vi "Manipulate frame size.vi"(8 "error in (no error)":errorcluster, 10 "Value":u16, 11 "Frame Size":refnum<vi>) -> (0 "error out":errorcluster, 3 "Updated frame size":T1=200 items=["100X100"=100, "128X128"=128, "200X200"=200, "256X256"=256, "512X512"=512, "1024x1024"=1024, "2048x2048"=2048])   [LabVIEW 2020]
uses:
  Typedefs/Frame Size.ctl
  3abac306-aade-448e-83a5-8b61187ab33a.vi
  <vilib>/Comparison/Equal/Equal Functor/Equal Functor.lvclass
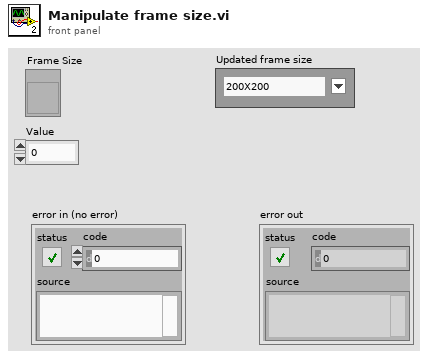
[diagram p1: front panel]
types:
  T1 = typedef "Frame Size.ctl" = u16
  T2 = typedef "LVStringsAndValuesArrayTypeDef_U16.ctl" = cluster{"String":string, "Value":u16}[]
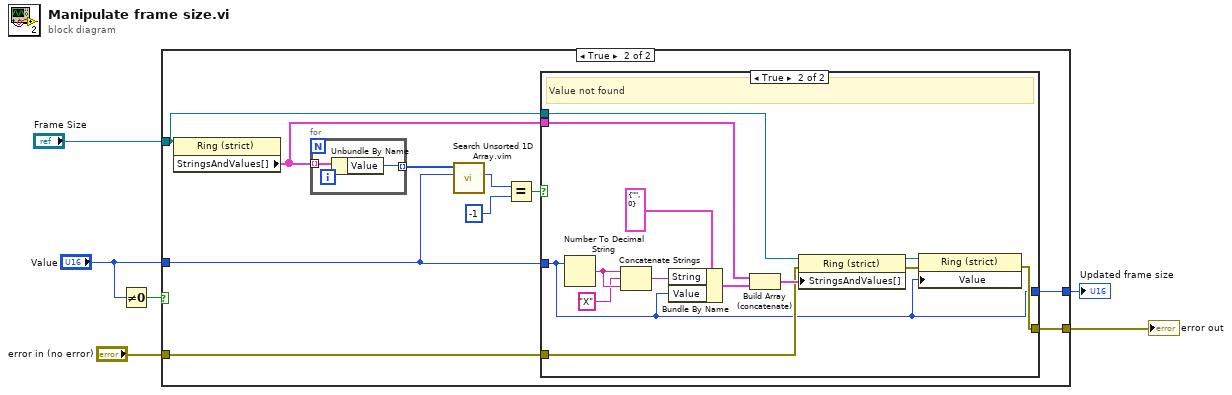
[diagram p0: block diagram]
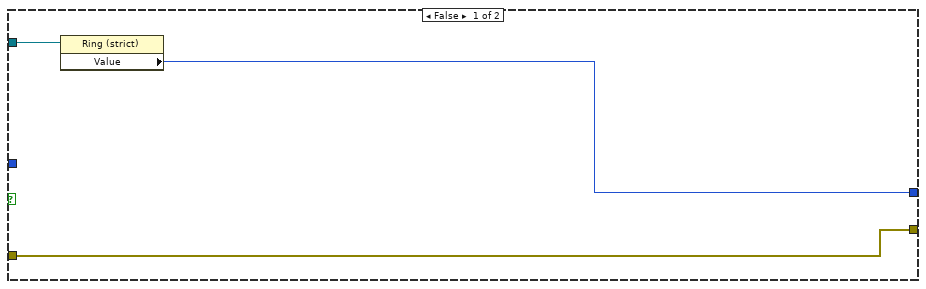
[diagram p2: hidden frame]
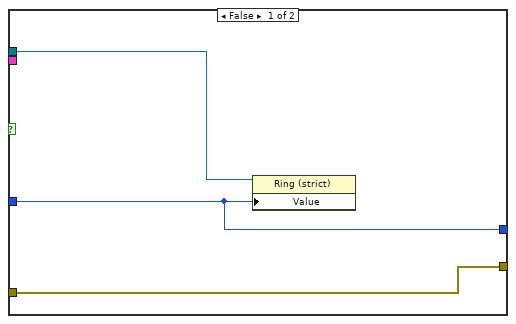
[diagram p3: hidden frame]
diagram:
  n1 = Not Equal To 0?(x="Value") -> (x != 0?=w4:bool)
  n2 = case shown="True" w4 {
    tunnel: "Frame Size" -> [w8 w13]
    tunnel: "Value" -> [_ w15]
    tunnel: "error in (no error)" -> [w9 w12]
    tunnel: [w9 w11] -> w2
    tunnel: [w7 w10] -> w1
    frame False {
      n3 = property class="Ring (strict)"(reference=w8) -> ("Value"=w7:T1)  [unwired: 1 in, 2 out]
    }
    frame True {
      n4 = property class="Ring (strict)"(reference=w13) -> ("StringsAndValues[]"=w14:T2)  [unwired: 1 in, 2 out]
      n5 = for {
        tunnel: w14 -> [w37] mode=indexing
        tunnel: [w36] -> w19 mode=indexing
        n6 = Unbundle By Name(w37) -> ("Value"=w36:u16)
      }
      n7 = call "Search Unsorted 1D Array.vim"("element"=w15, "unsorted 1D array"=w19) -> ("index of element"=w18:i32)  [unwired: 9 in]
      n8 = Equal?(x=w18, y=-1) -> (x = y?=w16:bool)
      n9 = case shown="True" w16 {
        tunnel: w15 -> [w20 w23]
        tunnel: w14 -> [_ w30]
        tunnel: w13 -> [w22 w28]
        tunnel: w12 -> [w21 w26]
        tunnel: [w21 w24] -> w11
        tunnel: [w20 w23] -> w10
        frame False {
          n10 = property class="Ring (strict)"(reference=w22, "Value"=w20) -> ()  [unwired: 1 in, 2 out]
        }
        frame True {
          # "Value not found"
          n11 = Number To Decimal String(number=w23) -> (decimal integer string=w35:string)  [unwired: 1 in]
          n12 = Concatenate Strings(w35, "X", w35) -> (w32:string)
          n13 = Bundle By Name(cluster=cluster{"String":string, "Value":u16} {"String"="", "Value"=0} ("Cluster"), "String"=w32, "Value"=w23) -> (w31:cluster{"String":string, "Value":u16})
          n14 = Build Array (concatenate)(w30, w31) -> (w29:T2)
          n15 = property class="Ring (strict)"(reference=w28, error in=w26, "StringsAndValues[]"=w29) -> (reference out=w27:refnum<vi>, error out=w25:errorcluster)
          n16 = property class="Ring (strict)"(reference=w27, error in=w25, "Value"=w23) -> (error out=w24:errorcluster)  [unwired: 1 out]
        }
      }
    }
  }
  "error out" <- w2
  "Updated frame size" <- w1
